vi "Get Config Directory Path.vi"() -> (3 "appended path":path)   [LabVIEW 2020, in "Utilities.lvlib"]
uses:
  Utilities.lvlib
  <vilib>/Utility/sysdir.llb/System Directory Type.ctl
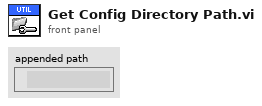
[diagram p1: front panel]
types:
  T1 = typedef "System Directory Type.ctl" = i32
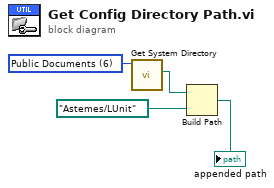
[diagram p0: block diagram]
diagram:
  w3 = T1 6 items=["User Home"=0, "User Desktop"=1, "User Documents"=2, "User Application Data"=3, "User Preferences"=4, "User Temporary"=5, "Public Documents"=6, "Public Application Data"=7, "Public Preferences"=8, "Public Cache"=13, "System Core Libraries"=9, "System Installed Libraries"=10, "Application Files"=11, "Boot Volume Root"=12] ("system directory type")
  n1 = call <vilib>:"Get System Directory.vi"("system directory type"=w3) -> ("system directory"=w1:path)  [unwired: 10 in]
  n2 = Build Path(base path=w1, name or relative path=path "Astemes/LUnit") -> (appended path=→"appended path":path)
